vi "Get SysDef Root Node IDs (SubVI).vi"(8 "error in (no error)":errorcluster, 11 "SysDef Refnum In":refnum<k39>) -> (0 "error out":errorcluster, 2 "Root NodeIDs Out":u64[](array[numeric]), 3 "SysDef Refnum Out":refnum<k39>)   [LabVIEW 2026, in "FPGA Addon Test Class.lvclass"]
uses:
  FPGA Addon Test Class.lvclass
  C:/Users/Administrator/Desktop/Jatin/All DNC DLLs/NationalInstruments.VeriStand.SystemDefinitionAPI.dll
  Jatin/All DNC DLLs/NationalInstruments.VeriStand.SystemDefinitionAPI.dll
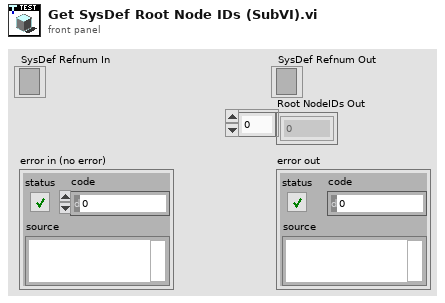
[diagram p1: front panel]
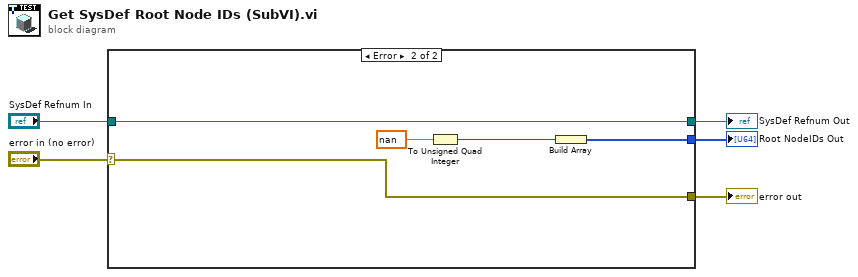
[diagram p0: block diagram]
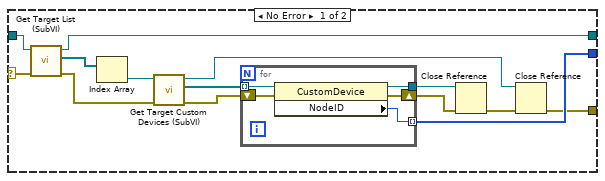
[diagram p2: hidden frame]
diagram:
  n1 = case shown="Error" "error in (no error)" {
    selector: "error in (no error)" -> [w14 w29]
    tunnel: [w8 w29] -> w5
    tunnel: "SysDef Refnum In" -> [w15 w26]
    tunnel: [w13 w25] -> w2
    tunnel: [w12 w26] -> w1
    frame No Error {
      n2 = call "Get Target List (SubVI).vi"("error in (no error)"=w14, "NationalInstruments.VeriStand.SystemDefinitionAPI.SystemDefinition"=w15) -> ("error out"=w18:errorcluster, "Target List Refnums"=w16:refnum<k39>[], "NationalInstruments.VeriStand.SystemDefinitionAPI.SystemDefinition"=w12:refnum<k39>)  [unwired: 7 in]
      n3 = Index Array(array=w16) -> (element=w17:refnum<k39>)  [unwired: 1 in]
      n4 = call "Get Target Custom Devices (SubVI).vi"("error in (no error)"=w18, "NationalInstruments.VeriStand.SystemDefinitionAPI.Target"=w17) -> ("error out"=w19:errorcluster, "Custom Devices Refnums"=w6:refnum<k39>[], "NationalInstruments.VeriStand.SystemDefinitionAPI.Target"=w7:refnum<k39>)  [unwired: 6 in, 1 out]
      n5 = for {
        tunnel: [w23] -> w13 mode=indexing
        tunnel: [w21] -> w10
        shift-right: [w22] -> w11
        shift-left: w19 -> [w24]
        tunnel: w6 -> [w20] mode=indexing
        n6 = property class="CustomDevice"(reference=w20, error in=w24) -> (reference out=w21:refnum<k39>, error out=w22:errorcluster, "NodeID"=w23:u64)
      }
      n7 = Close Reference(reference=w10, error in (no error)=w11) -> (error out=w9:errorcluster)
      n8 = Close Reference(reference=w7, error in (no error)=w9) -> (error out=w8:errorcluster)
    }
    frame Error {
      n9 = To Unsigned Quad Integer(1:nan) -> (0:w27:u64)
      n10 = Build Array(w27) -> (w25:u64[])
    }
  }
  "error out" <- w5
  "Root NodeIDs Out" <- w2
  "SysDef Refnum Out" <- w1
